vi "GB_Remote Sense Test_v2.vi"(7 "error in (no error)":errorcluster, 9 "HMP VISA":refnum<visa-resource-name>, 10 "ControlBoard VISA":refnum<visa-resource-name>="ControlBoard") -> (0 "error out":errorcluster, 2 "Voltage Readings":dbl[][](array[numeric]), 3 "Pass?":bool)   [LabVIEW 2022 SP3]
uses:
  HMP4040_ChannelControlAutomatic.ctl
panel:
  out "Message OUT":string
  out "MSE Array":dbl[](array[numeric])
  in  "Message IN":string
  out "Control Board OUT":refnum<visa-resource-name>
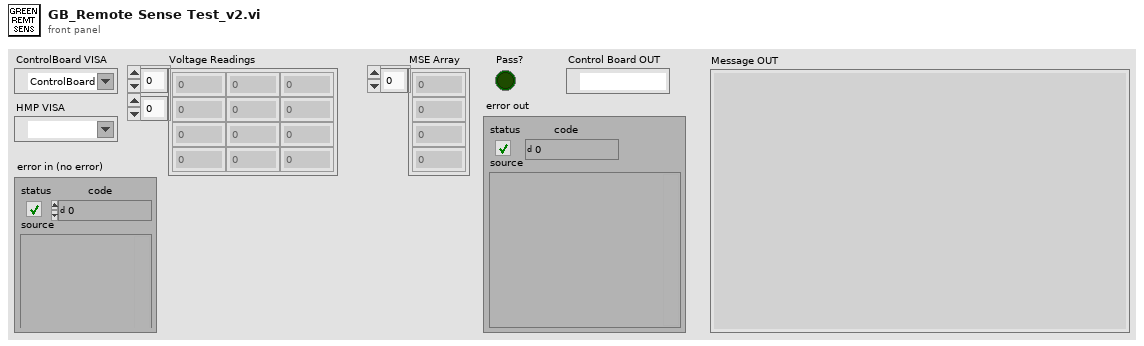
[diagram p1: front panel]
types:
  T1 = typedef "HMP4040_ChannelControlAutomatic.ctl" = enum16{"Off", "Control Power", "HMP2020 Control + DC32V", "HMP2020 Control + DC8V", "HMP4040 Control + DC32V", "HMP4040 Control +DC8V", "HMP4040 Ch2 24V 4A"}
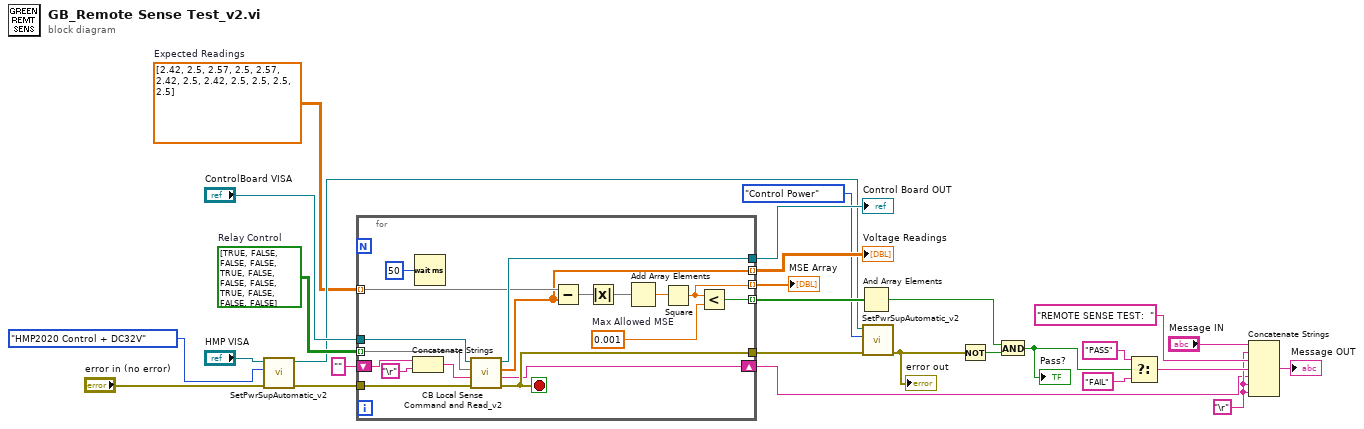
[diagram p0: block diagram]
diagram:
  w1 = dbl[][] [[2.42, 2.5, 2.57], [2.5, 2.57, 2.42], [2.5, 2.42, 2.5], [2.5, 2.5, 2.5]]  # Expected Readings
  w15 = "\r"
  w25 = bool[][] [[TRUE, FALSE, FALSE], [FALSE, TRUE, FALSE], [FALSE, FALSE, TRUE], [FALSE, FALSE, FALSE]]  # Relay Control
  n1 = call "SetPwrSupAutomatic_v2.vi"("error in (no error)"="error in (no error)", "Enum"=HMP4040_ChannelControlAutomatic."HMP2020 Control + DC32V", "HMP VISA"="HMP VISA") -> ("error out"=w3:errorcluster, "HMP VISA Out"=w5:refnum<visa-resource-name>)  [unwired: 7 in]
  n2 = for {
    tunnel: [w43] -> w6
    tunnel: [w45] -> w27
    tunnel: w3 -> [w44]
    tunnel: w1 -> [w40] mode=indexing
    tunnel: [w37] -> w26 mode=indexing
    tunnel: w25 -> [w36] mode=indexing
    tunnel: [w35] -> w22 mode=indexing
    tunnel: [w34] -> w21 mode=indexing
    shift-right: [w33] -> w13
    shift-left: "" -> [w32]
    tunnel: "ControlBoard VISA" -> [w28]
    stop <- w43 stop-if-true
    w38 = 0.001  # Max Allowed MSE
    n3 = Concatenate Strings(w32, "\r") -> (w31:string)
    n4 = Wait (ms)(milliseconds to wait=u32 50) -> ()  [unwired: 1 out]
    n5 = call "CB Local Sense Command and Read_v2.vi"("error in (no error)"=w44, "Message IN"=w31, "Relay Control"=w36, "Control Board VISA"=w28) -> ("error out"=w43:errorcluster, "Message OUT"=w33:string, "Voltage Array"=w35:dbl[], "Control Board OUT"=w45:refnum<visa-resource-name>)  [unwired: 4 in]
    n6 = Subtract(x=w40, y=w35) -> (x-y=w42:dbl[])
    n7 = Absolute Value(x=w42) -> (abs(x)=w41:dbl[])
    n8 = Add Array Elements(numeric array=w41) -> (sum=w39:dbl)
    n9 = Square(x=w39) -> (x^2=w34:dbl)
    n10 = Less?(x=w34, y=w38) -> (x < y?=w37:bool)
  }
  "Voltage Readings" <- w22
  "MSE Array" <- w21
  "Control Board OUT" <- w27
  n11 = And Array Elements(Boolean array=w26) -> (logical AND=w24:bool)
  n12 = call "SetPwrSupAutomatic_v2.vi"("error in (no error)"=w6, "Enum"=HMP4040_ChannelControlAutomatic."Control Power", "HMP VISA"=w5) -> ("error out"=w7:errorcluster)  [unwired: 7 in, 1 out]
  "error out" <- w7
  n13 = Not(x=w7) -> (.not. x?=w23:bool)
  n14 = And(x=w24, y=w23) -> (x .and. y?=w14:bool)
  "Pass?" <- w14
  n15 = Select(t="PASS", s=w14, f="FAIL") -> (s? t:f=w19:string)
  n16 = Concatenate Strings("Message IN", w15, "REMOTE SENSE TEST:  ", w19, w13, w15, w15) -> (→"Message OUT":string)
